vi "VNA Initialize - SParam.vi"(8 "error in":errorcluster, 10 "RFmxVNA Settings":T1={"Resource Name"="", "vCal Name"="", "RFmxVNA Calset Enable"=FALSE, "RFmxVNA Calset Interpolation"=FALSE, "Calset File Path"="", "RFmxVNA attenuation mode"=enum."s2p File", "RFmxVNA Port1 s2p file path"="", "RFmxVNA Port1 s-parameters orientation"=enum."Port1 Towards DUT", "RFmxVNA Port1 Power Compensation"=FALSE, "RFmxVNA Port2 s2p file path"="", "RFmxVNA Port2 s-parameters orientation"=enum."Port1 Towards DUT", "RFmxVNA Port2 Power Compensation"=FALSE, "Port1 Power Level (dBm)"=0.0, "Port1 Test Receiver Attenuation (dB)"=0.0, "Port2 Power Level (dBm)"=0.0, "Port2 Test Receiver Attenuation (dB)"=0.0, "IF Bandwidth (Hz)"=0.0, "Frequency Sweep"={"Start Frequency (Hz)"=4000000000.0, "Stop Frequency (Hz)"=26000000000.0, "Number of Points"=200}} {"Frequency Sweep"."Stop Frequency (Hz)" format="%.3p"; "Frequency Sweep"."Start Frequency (Hz)" format="%.3p"; "IF Bandwidth (Hz)" format="%.2p"; "Port2 Test Receiver Attenuation (dB)" format="%.2f"; "Port2 Power Level (dBm)" format="%.2f"; "Port1 Test Receiver Attenuation (dB)" format="%.2f"; "Port1 Power Level (dBm)" format="%.2f"}) -> (0 "error out":errorcluster, 3 "RFmxVNA Session out":refnum<k21>)   [LabVIEW 2023]
uses:
  Controls/RFmxVNA Config - SParam.ctl
  <vilib>/RFmx/VNA/mx/RFmxVNA.llb/RFmxVNA Select Measurement (Single).vi
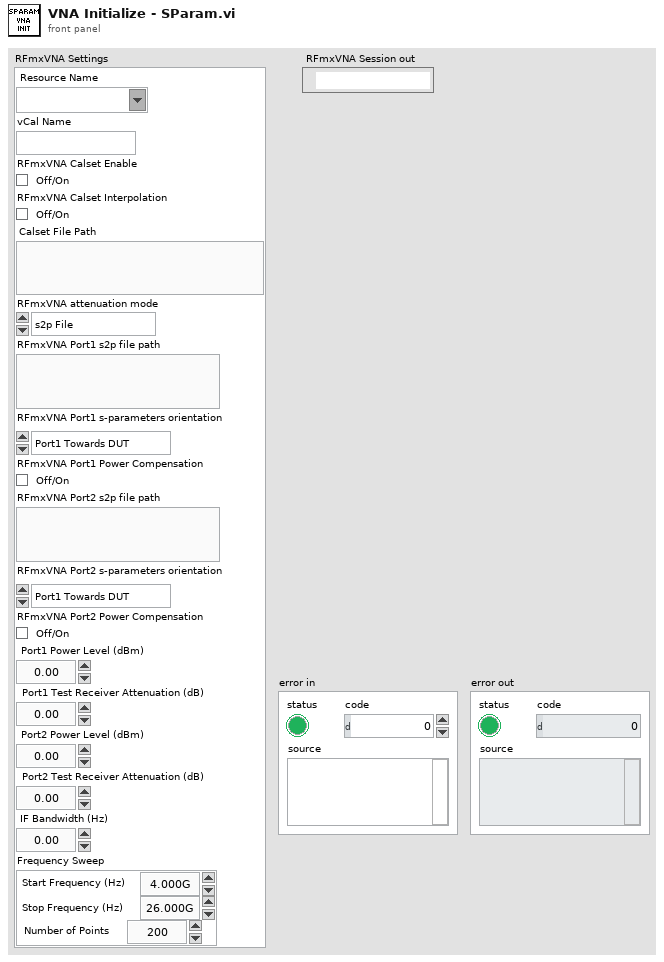
[diagram p1: front panel]
types:
  T1 = typedef "RFmxVNA Config - SParam.ctl" = cluster{"Resource Name":refnum<k15>, "vCal Name":string, "RFmxVNA Calset Enable":bool, "RFmxVNA Calset Interpolation":bool, "Calset File Path":string, "RFmxVNA attenuation mode":enum32{"<None>", "s2p File"}, "RFmxVNA Port1 s2p file path":string, "RFmxVNA Port1 s-parameters orientation":enum32{"Port1 Towards DUT", "Port2 Towards DUT"}, "RFmxVNA Port1 Power Compensation":bool, "RFmxVNA Port2 s2p file path":string, "RFmxVNA Port2 s-parameters orientation":enum32{"Port1 Towards DUT", "Port2 Towards DUT"}, "RFmxVNA Port2 Power Compensation":bool, "Port1 Power Level (dBm)":dbl, "Port1 Test Receiver Attenuation (dB)":dbl, "Port2 Power Level (dBm)":dbl, "Port2 Test Receiver Attenuation (dB)":dbl, "IF Bandwidth (Hz)":dbl, "Frequency Sweep":cluster{"Start Frequency (Hz)":dbl, "Stop Frequency (Hz)":dbl, "Number of Points":i32}}
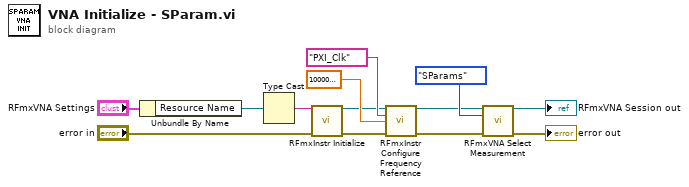
[diagram p0: block diagram]
diagram:
  n1 = Unbundle By Name("RFmxVNA Settings") -> ("Resource Name"=w6:refnum<k15>)
  n2 = Type Cast(x=w6) -> (*(type *) &x=w11:string)  [unwired: 1 in]
  n3 = call <vilib>:"RFmxInstr Initialize.vi"("Resource Name"=w11, "error in (no error)"="error in") -> ("Instrument Handle Out"=w8:refnum<k21>, "error out"=w7:errorcluster)  [unwired: 11 in, 1 out]
  n4 = call <vilib>:"RFmxInstr Configure Frequency Reference.vi"("Instrument Handle In"=w8, "Frequency Reference Source"="PXI_Clk" ("Frequency Source"), "Frequency (Hz)"=100000000.0, "error in (no error)"=w7) -> ("Instrument Handle Out"=w2:refnum<k21>, "error out"=w1:errorcluster)  [unwired: 10 in]
  n5 = call-poly <vilib>:"RFmxVNA Select Measurement.vi"("Instrument Handle In"=w2, "Measurement"=enum16{"SParams", "Waves", "IQ"}."SParams", "error in (no error)"=w1) -> ("Instrument Handle Out"=→"RFmxVNA Session out":refnum<k21>, "error out"=→"error out":errorcluster)  [unwired: 11 in]
